vi "TSM SSC Digital Frequency Counter Measure Frequency.vi"(0 "Digital TSM In":T1, 11 "error in":errorcluster) -> (4 "Digital TSM Out":T1, 6 "Per-Site Per-Pin Frequency Measurements (Hz)":dbl[][](array[numeric]), 15 "error out":errorcluster)   [LabVIEW 2020]
doc: "Measures the frequency on the specified pin(s) and pin group(s) over the configured measurement time and returns per-site frequency measurements."
uses:
  TSM/TSM SSC Digital.ctl
  <vilib>/NI_TestStand_SemiconductorModule/NI_TestStand_Semiconductor_Module.lvlibp/PinMap/Digital Pattern/PinQueryContext/DigitalPatternPinQueryContext.lvclass
  SSC Digital/SSC Digital.ctl
  d407e431-de4a-4cf0-a152-125e2a403964.vi
  Shared SubVIs/Channel List to Pins.vi
  Shared SubVIs/Trim Whitespace [Inlined].vi
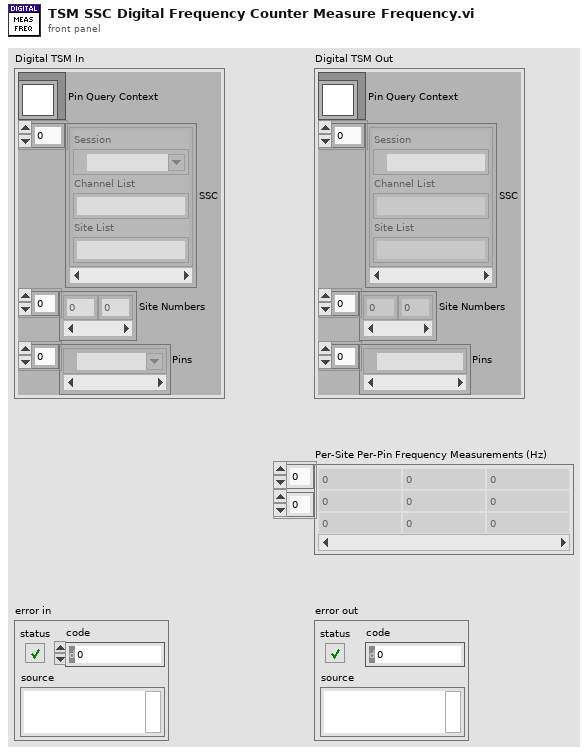
[diagram p1: front panel]
types:
  T1 = typedef "TSM SSC Digital.ctl" = cluster{"Pin Query Context":refnum<class "DigitalPatternPinQueryContext.lvclass">, "SSC":T2[], "Site Numbers":i32[], "Pins":tag[]}
  T2 = typedef "SSC Digital.ctl" = cluster{"Session":refnum<k15>, "Channel List":string, "Site List":string}
  T3 = typedef "Digital 2D Location Array in a Cluster.ctl" = cluster{"Digital 2D Location Array":T4[]}
  T4 = typedef "Digital 2D Location.ctl" = cluster{"Row":i32, "Col":i32}
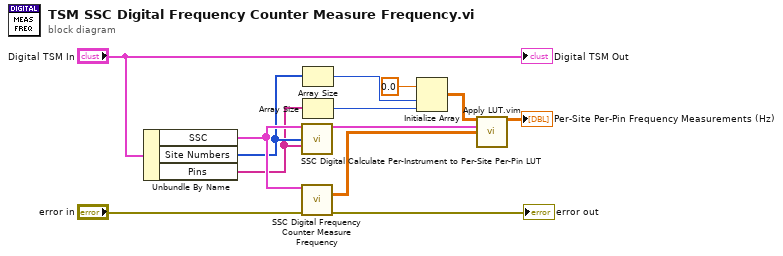
[diagram p0: block diagram]
diagram:
  n1 = Unbundle By Name("Digital TSM In") -> ("SSC"=w7:T2[], "Site Numbers"=w6:i32[], "Pins"=w2:tag[])
  n2 = call "SSC Digital Calculate Per-Instrument to Per-Site Per-Pin LUT.vi"("Digital SSC In"=w7, "Sites"=w6, "Pins"=w2) -> ("Per-Instrument to Per-Site Per-Pin LUT"=w11:T3[])  [unwired: 12 in]
  n3 = call "SSC Digital Frequency Counter Measure Frequency.vi"("Digital SSC in"=w7, "error in"="error in") -> ("Per-Instrument Frequencies (Hz)"=w4:dbl[][], "error out"=→"error out":errorcluster)  [unwired: 11 in, 1 out]
  n4 = Array Size(array=w6) -> (size(s)=w10:i32)
  n5 = Array Size(array=w2) -> (size(s)=w1:i32)
  n6 = Initialize Array(0.0, w10, w1) -> (w8:dbl[][])
  n7 = call "Apply LUT.vim"("Initialized Array"=w8, "LUT"=w11, "Results to Apply LUT to"=w4) -> ("Array Out"=→"Per-Site Per-Pin Frequency Measurements (Hz)":dbl[][])  [unwired: 12 in]
  "Digital TSM Out" <- "Digital TSM In"
